vi "Fit.vi"(8 "error in (no error)":errorcluster caption="entrée d'erreur (pas d'erreur)", 9 "y":string[][](array[string]), 10 "X":string[][](array[string]), 11 "FeatureHasher.lvclass":refnum<class "FeatureHasher.lvclass">) -> (0 "error out":errorcluster caption="sortie d'erreur", 2 "String Data":string, 3 "FeatureHasher.lvclass":refnum<class "FeatureHasher.lvclass">)   [LabVIEW 2020, in "FeatureHasher.lvclass"]
doc: "No-op.\n\nThis method doesn’t do anything. It exists purely for compatibility with the scikit-learn transformer API.\n\nReturns :\n\n- String : OK"
uses:
  FeatureHasher.lvclass
  FeatureHasher.lvclass/FeatureHasher.ctl
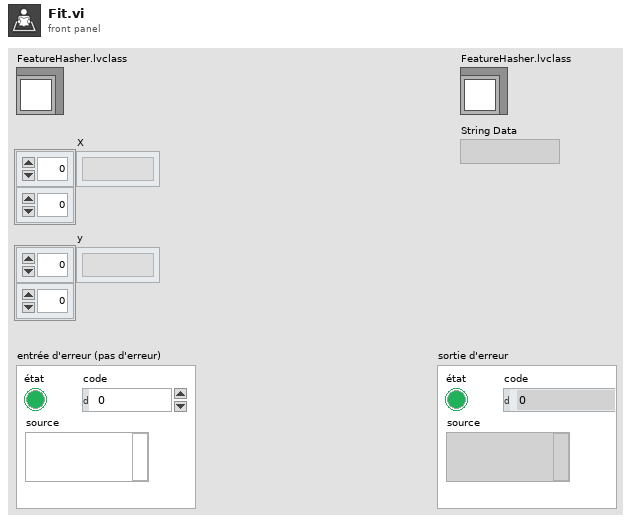
[diagram p1: front panel]
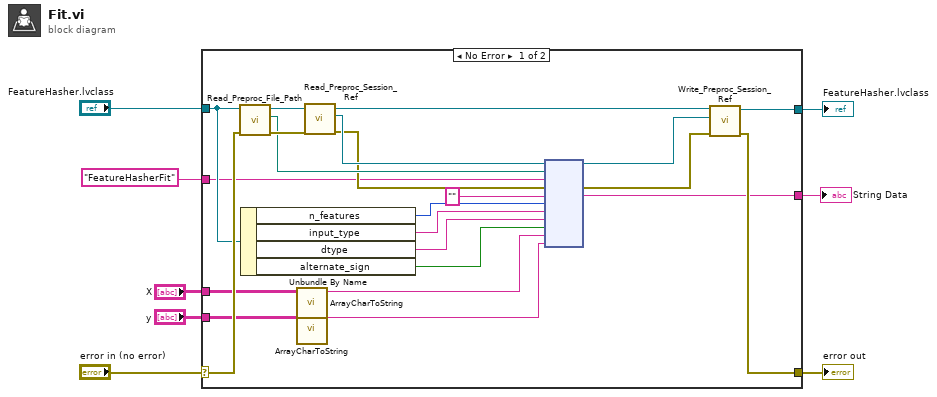
[diagram p0: block diagram]
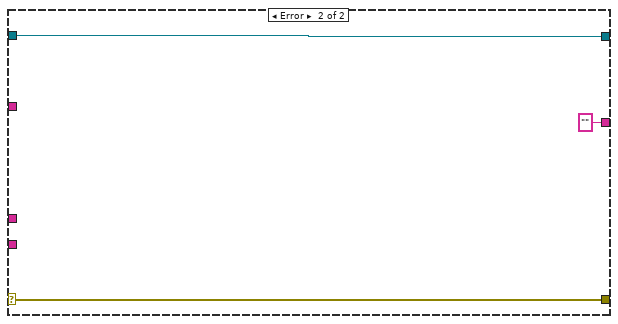
[diagram p2: hidden frame]
diagram:
  n1 = case shown="No Error" "error in (no error)" {
    selector: "error in (no error)" -> [w18 w34]
    tunnel: [w17 w34] -> w7
    tunnel: [w19 w33] -> w5
    tunnel: "FeatureHasher.lvclass" -> [w16 w33]
    tunnel: "FeatureHasherFit" ("Fonction") -> [w15 _]
    tunnel: "X" -> [w12 _]
    tunnel: [w14 ""] -> w2
    tunnel: "y" -> [w10 _]
    frame No Error {
      n2 = call-dynamic "Read_Preproc_File_Path.vi"("error in (no error)"=w18, "Python in"=w16) -> ("error out"=w30:errorcluster, "File_Path"=w29:path, "Python out"=w31:refnum<class "FeatureHasher.lvclass">)  [unwired: 7 in]
      n3 = Unbundle By Name(w16) -> ("n_features"=w22:i32, "input_type"=w21:string, "dtype"=w20:string, "alternate_sign"=w13:bool)
      n4 = call "ArrayCharToString.vi"("TAB"=w12) -> ("Instruction"=w11:string)  [unwired: 10 in]
      n5 = call "ArrayCharToString.vi"("TAB"=w10) -> ("Instruction"=w9:string)  [unwired: 10 in]
      n6 = call-dynamic "Read_Preproc_Session_Ref.vi"("error in (no error)"=w30, "Python in"=w31) -> ("error out"=w27:errorcluster, "Session_ref"=w28:refnum<k35>, "Python out"=w26:refnum<class "FeatureHasher.lvclass">)  [unwired: 7 in]
      n7 = node(w28, w29, w15, w27, "", w22, w21, w20, w13, w11, w9) -> (w24:refnum<k35>, w25:errorcluster, w14:string)  [unwired: 6 in, 2 out]
      n8 = call-dynamic "Write_Preproc_Session_Ref.vi"("error in (no error)"=w25, "Session_ref"=w24, "Python in"=w26) -> ("error out"=w17:errorcluster, "Python out"=w19:refnum<class "FeatureHasher.lvclass">)  [unwired: 7 in]
    }
    frame Error {
    }
  }
  "error out" <- w7
  "FeatureHasher.lvclass" <- w5
  "String Data" <- w2
